vi "OFDMwithTextRX.vi"() -> ()   [LabVIEW 2022 SP3]
uses:
  <vilib>/Analysis/2dsp.llb/Complex FFT.vi
  <instrlib>/niUSRP/niUSRP Fetch Rx Data (CDB).vi
  <vilib>/addons/Modulation/Digital/General/MT Map QAM Symbols to Bits.vi
  <vilib>/Analysis/NI_AALPro.lvlib
  <vilib>/addons/Modulation/niDMT.lvlib
panel:
  out "output string":string
  out "output bit stream":i8[][](array[numeric]) format="%b"
  in  "Tab Control":enum32{"Parameters", "Debug", "CFO"}(tab)
  in  "Device names":refnum<k15>="192.168.10.3"
  in  "Active antenna":string="RX1"
  in  "Gain":dbl=3.0 format="%#_6f"
  in  "Carrier frequency":dbl=910000000.0 format="%#_6p"
  in  "IQ rate":dbl=5000000.0 format="%#_6p"
  in  "Number of samples":i64=1600
  out "Coerced IQ rate":dbl=100000.0 format="%#_6p"
  in  "stop":bool
  out "Output bit stream":i8[](array[numeric]) caption="output bit stream"
  out "error out":errorcluster
  out "error out 2":errorcluster
  out "CFOest (Hz)":dbl[](array[numeric])
  out "Equalized Data":cdb[](graph)
  out "Unequalized Data":cdb[](graph)
  out "theta":dbl[](graph)
  out "FFT {X}":dbl[](graph)
  out "Phase":dbl[](graph)
  out "Magnitude":dbl[](graph)
  # "OFDM Receiver"
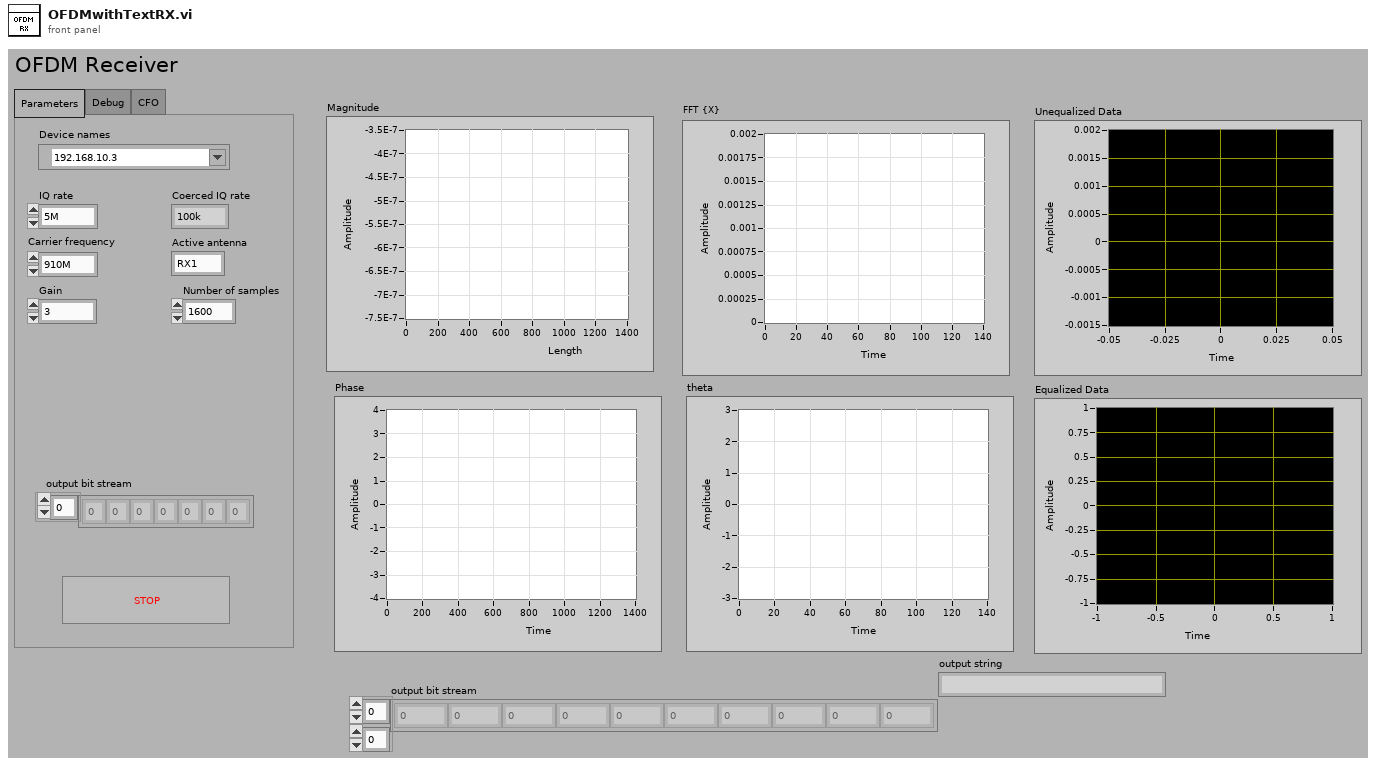
[diagram p1: front panel]
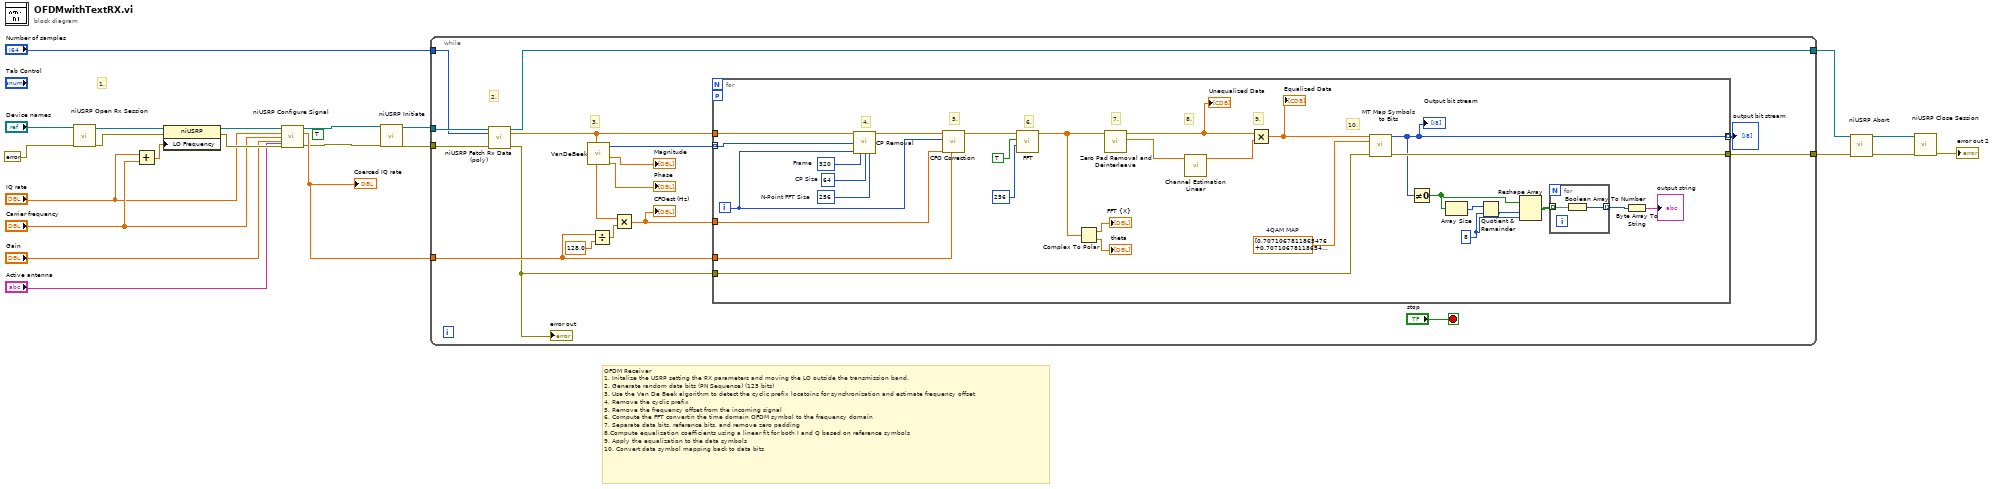
[diagram p0: block diagram]
diagram:
  (unwired) TRUE ("number of samples is finite")
  # "1."
  # "OFDM Receiver\n1. Initalize the USRP setting the RX parameters and moving the LO outside the transmission band.\n2. Generate random data bits (PN Sequence) (125 bits)\n3. Use the Van De Beek algorithm to detect the cyclic prefix locatoins for synchronization and estimate frequency offset\n4. Remove the cyclic prefix\n5. Remove the frequency offset from the incoming signal\n6. Compute the FFT convertin the time domain OFDM symbol to the frequency domain\n7. Separate data bits, reference bits, and remove zero padding\n8.Compute equalization coefficients using a linear fit for both I and Q based on reference symbols \n9. Apply the equalization to the data symbols\n10. Convert data symbol mapping back to data bits"
  n1 = call <instrlib>:"niUSRP Open Rx Session.vi"("device names"="Device names", "error in (no error)"=errorcluster {"status"=FALSE, "code"=0, "source"=""}) -> ("session handle out"=w20:refnum<k15>, "error out"=w18:errorcluster)  [unwired: 12 in]
  n2 = Add(x="IQ rate", y="Carrier frequency") -> (x+y=w12:dbl)
  n3 = property class="niUSRP"(reference=w20, error in=w18, "LO Frequency"=w12) -> (reference out=w19:refnum<k15>, error out=w17:errorcluster)
  n4 = call <instrlib>:"niUSRP Configure Signal.vi"("session handle"=w19, "IQ rate"="IQ rate", "carrier frequency"="Carrier frequency", "gain"="Gain", "error in (no error)"=w17, "active antenna"="Active antenna") -> ("session handle out"=w2:refnum<k15>, "coerced IQ rate"=w3:dbl, "error out"=w1:errorcluster)  [unwired: 5 in, 2 out]
  "Coerced IQ rate" <- w3
  n5 = call <instrlib>:"niUSRP Initiate.vi"("session handle"=w2, "error in (no error)"=w1) -> ("session handle out"=w22:refnum<k15>, "error out"=w21:errorcluster)  [unwired: 12 in]
  n6 = while {
    tunnel: w22 -> [w36]
    tunnel: w21 -> [w31]
    tunnel: [w35] -> w6
    tunnel: "Number of samples" -> [w32]
    tunnel: w3 -> [w38]
    tunnel: [w37] -> w9
    stop <- "stop" stop-if-true
    # "2."
    # "3."
    n7 = call-poly <instrlib>:"niUSRP Fetch Rx Data (poly).vi"("session handle"=w36, "number of samples"=w32, "error in (no error)"=w31) -> ("session handle out"=w35:refnum<k15>, "data"=w33:cdb[], "error out"=w34:errorcluster)  [unwired: 9 in, 1 out]
    "error out" <- w34
    n8 = call "VanDeBeek.vi"("Input"=w33) -> ("Phase"=→"Phase":dbl[], "Magnitude"=→"Magnitude":dbl[], "Indices"=w28:i32[], "CFOest (Hz)"=w27:dbl[])  [unwired: 6 in, 1 out]
    n9 = Divide(x=w38, y=128.0 ("x")) -> (x/y=w29:dbl)
    n10 = Multiply(x=w27, y=w29) -> (x*y=w24:dbl[])
    "CFOest (Hz)" <- w24
    n11 = for {
      tunnel: w24 -> [w61]
      workers-P: _ -> [_]
      tunnel: w38 -> [w60]
      tunnel: w34 -> [w59]
      tunnel: [w58] -> w37
      tunnel: w28 -> [w53] mode=indexing
      tunnel: w33 -> [w56]
      tunnel: [w47] -> w23 mode=indexing
      i -> [w51]
      w43 = 8 ("y")
      w52 = 256  # N-Point FFT Size
      w55 = 64  # CP Size
      w63 = cdb[] [0.7071067811865476+0.7071067811865476i, 0.7071067811865476-0.7071067811865476i, -0.7071067811865476+0.7071067811865476i, -0.7071067811865476-0.7071067811865476i]  # 4QAM MAP
      w54 = 320  # Frame
      # "10."
      # "9."
      # "8."
      # "7."
      # "6."
      # "5."
      # "4."
      n12 = call "CP Removal.vi"("Input"=w56, "Indicies"=w53, "i"=w51, "Frame Size"=w54, "CP Size"=w55, "N-Point FFT Size"=w52) -> ("Output Without CP"=w57:cdb[])  [unwired: 9 in]
      n13 = call "CFO Correction.vi"("fs"=w60, "CFOest (freq)"=w61, "Index"=w51, "Input"=w57) -> ("Output"=w64:cdb[])  [unwired: 7 in]
      n14 = call-poly <vilib>:"FFT.vi"("FFT size"=256, "shift?"=TRUE, "X"=w64) -> ("FFT {X}"=w65:cdb[])  [unwired: 7 in, 1 out]
      n15 = Complex To Polar(r * e^(i*theta)=w65) -> (r=→"FFT {X}":dbl[], theta=→"theta":dbl[])
      n16 = call "Zero Pad Removal and Deinterleave.vi"("Input"=w65) -> ("Ref"=w50:cdb[], "Data"=w48:cdb[])  [unwired: 9 in]
      "Unequalized Data" <- w48
      n17 = call "Channel Estimation Linear.vi"("Ref"=w50) -> ("Hest"=w49:cdb[])  [unwired: 10 in]
      n18 = Multiply(x=w48, y=w49) -> (x*y=w62:cdb[])
      "Equalized Data" <- w62
      n19 = call-poly <vilib>:"MT Map Symbols to Bits.vi"("symbols"=w62, "symbol map"=w63, "error in (no error)"=w59) -> ("output bit stream"=w47:i8[], "error out"=w58:errorcluster)  [unwired: 11 in]
      "Output bit stream" <- w47
      n20 = Not Equal To 0?(x=w47) -> (x != 0?=w45:bool[])
      n21 = Array Size(array=w45) -> (size(s)=w46:i32)
      n22 = Quotient & Remainder(x=w46, y=w43) -> (floor(x/y)=w44:i32)  [unwired: 1 out]
      n23 = Reshape Array(w45, w44, w43) -> (w42:bool[][])
      n24 = for {
        tunnel: w42 -> [w71] mode=indexing
        tunnel: [w70] -> w41 mode=indexing
        n25 = Boolean Array To Number(Boolean array=w71) -> (number=w70:u32)
      }
      n26 = Byte Array To String(unsigned byte array=w41) -> (string=→"output string":string)
    }
    "output bit stream" <- w23
  }
  n27 = call <instrlib>:"niUSRP Abort.vi"("session handle"=w6, "error in (no error)"=w9) -> ("session handle out"=w7:refnum<k15>, "error out"=w8:errorcluster)  [unwired: 12 in]
  n28 = call <instrlib>:"niUSRP Close Session.vi"("session handle"=w7, "error in (no error)"=w8) -> ("error out"=→"error out 2":errorcluster)  [unwired: 13 in]
